vi "append to file.vi"(2 "Analog Dataset":dbl[][](array[numeric])=[[34.0, 43.0, 0.0], [65.0, 44.0, 4.0], [4.0, 4.0, 12.0], [3.0, 22.0, 0.0]], 3 "Ring 2":u16(ring) items=["Dataset 1"=1, "Dataset 2"=2], 4 "Phase":string(combo), 5 "file path (use dialog)":path) -> (0 "error out":errorcluster, 1 "output string":string)   [LabVIEW 2021]
uses:
  <vilib>/Utility/file.llb/Write Delimited Spreadsheet (DBL).vi
panel:
  out "spreadsheet string":string
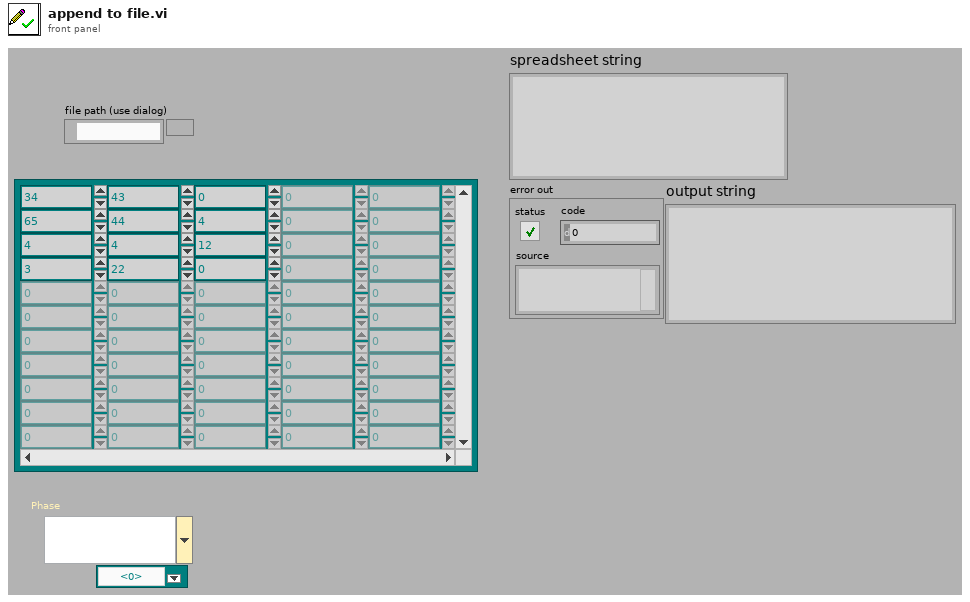
[diagram p1: front panel]
types:
  T1 = enum16{"open", "replace", "create", "open or create", "replace or create", "replace or create with confirmation"}
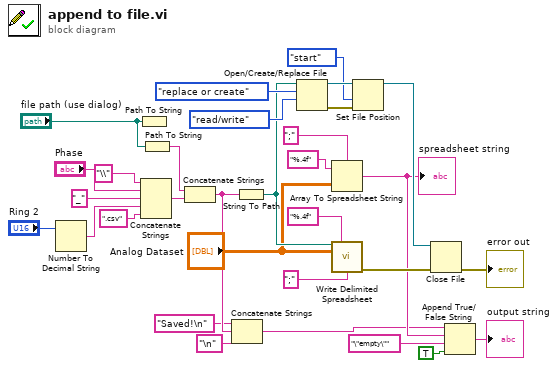
[diagram p0: block diagram]
diagram:
  n1 = Number To Decimal String(number="Ring 2") -> (decimal integer string=w6:string)  [unwired: 1 in]
  n2 = Path To String(path="file path (use dialog)") -> ()  [unwired: 1 out]
  n3 = Concatenate Strings("\\" ("string"), "Phase", "_" ("string"), w6, ".csv" ("string")) -> (w22:string)
  n4 = Path To String(path="file path (use dialog)") -> (string=w23:string)
  n5 = Concatenate Strings(w23, w22) -> (w4:string)
  n6 = Concatenate Strings("Saved!\n" ("string (\"\")"), w4, "\n" ("string")) -> (w2:string)
  n7 = String To Path(string=w4) -> (path=w19:path)
  n8 = Open/Create/Replace File(file path (use dialog)=w19, operation (0:open)=T1."replace or create", access (0:read/write)=enum16{"read/write", "read-only", "write-only"}."read/write") -> (refnum out=w29:refnum<file>, error out=w27:errorcluster)  [unwired: 3 in, 1 out]
  n9 = Array To Spreadsheet String(delimiter (Tab)=";", array="Analog Dataset", 3:"%.4f" ("format string")) -> (spreadsheet string=w12:string)
  "spreadsheet string" <- w12
  n10 = call-poly <vilib>:"Write Delimited Spreadsheet.vi"("file path (dialog if empty)"=w19, "format (%.3f)"="%.4f", "2D data"="Analog Dataset", "delimiter (\\t)"=";" ("delimiter (\\t)")) -> ("error out"=w20:errorcluster)  [unwired: 10 in, 1 out]
  n11 = Set File Position(refnum=w29, from (0:start)=enum16{"start", "end", "current"}."start", error in=w27) -> (refnum out=w18:refnum<file>)  [unwired: 1 in, 1 out]
  n12 = Close File(refnum=w18, error in=w20) -> (error out=→"error out":errorcluster)  [unwired: 1 out]
  n13 = Append True/False String(1:TRUE ("selector"), 2:"\"empty\"" ("false string"), 3:w12, 4:w2) -> (0:→"output string":string)
